vi "LV_DA转换 输出.vi"(9 "DA通道":i32=1 min=0 max=1, 10 "输入电压":dbl) -> ()   [LabVIEW 2010]
uses:
  idd.vi
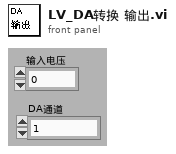
[diagram p1: front panel]
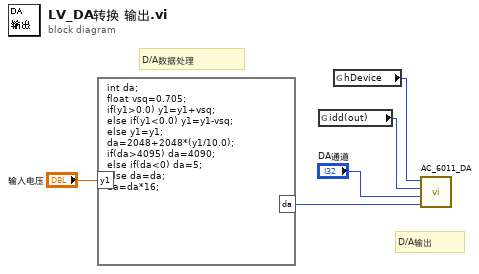
[diagram p0: block diagram]
diagram:
  # "D/A输出"
  # "D/A数据处理"
  n1 = formula code="int da;\nfloat vsq=0.705;\nif(y1>0.0) y1=y1+vsq;\nelse if(y1<0.0) y1=y1-vsq;\nelse y1=y1;\nda=2048+2048*(y1/10.0);\nif(da>4095) da=4090;\nelse if(da<0) da=5;\nelse da=da;\nda=da*16;"("y1"="输入电压") -> ("da"=w2:i32)
  n2 = global read "idd.vi" "idd(out)"() -> (w5:u32)
  n3 = global read "idd.vi" "hDevice"() -> (w3:u32)
  n4 = call "AC_6011_DA.vi"("DAData"=w2, "DAch"="DA通道", "idd(out)"=w5, "hDevice"=w3) -> ()  [unwired: 1 out]
